vi "Set Slew Rates.vi"(0 "instrument handle":refnum<visa-resource-name>, 1 "current slew rate":sgl, 2 "power slew rate":sgl, 3 "error in (no error)":errorcluster {"code" format="%.0x"}, 4 "voltage slew rate":sgl, 5 "resistance slew rate":sgl) -> (6 "instrument handle out":refnum<visa-resource-name>, 9 "error out":errorcluster {"code" format="%.0x"})   [LabVIEW 2018]
uses:
  <instrlib>/NHRDCPowerModule/NHRDCPowerModule/NHRDCPowerModule.lvlib
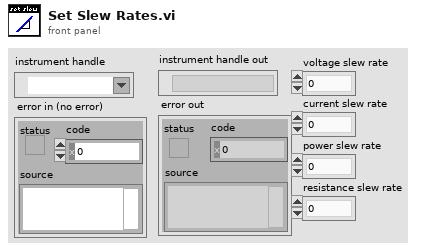
[diagram p1: front panel]
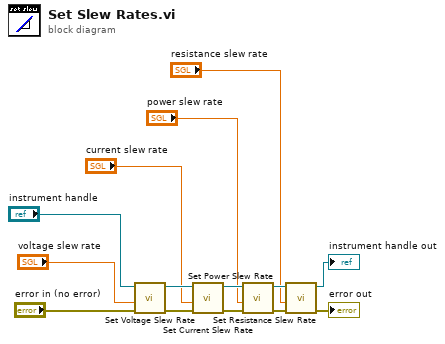
[diagram p0: block diagram]
diagram:
  n1 = call <instrlib>:"Set Voltage Slew Rate.vi"("error in (no error)"="error in (no error)", "voltage slew rate (0.0)"="voltage slew rate", "instrument handle"="instrument handle") -> ("error out"=w7:errorcluster, "instrument handle out"=w14:refnum<visa-resource-name>)  [unwired: 7 in]
  n2 = call <instrlib>:"Set Current Slew Rate.vi"("error in (no error)"=w7, "current slew rate (0.0)"="current slew rate", "instrument handle"=w14) -> ("error out"=w6:errorcluster, "instrument handle out"=w13:refnum<visa-resource-name>)  [unwired: 7 in]
  n3 = call <instrlib>:"Set Power Slew Rate.vi"("error in (no error)"=w6, "power slew rate (0.0)"="power slew rate", "instrument handle"=w13) -> ("error out"=w5:errorcluster, "instrument handle out"=w12:refnum<visa-resource-name>)  [unwired: 7 in]
  n4 = call <instrlib>:"Set Resistance Slew Rate.vi"("error in (no error)"=w5, "resistance slew rate (0.0)"="resistance slew rate", "instrument handle"=w12) -> ("error out"=→"error out":errorcluster, "instrument handle out"=→"instrument handle out":refnum<visa-resource-name>)  [unwired: 7 in]
